vi "octave_var.vi"() -> ()   [LabVIEW 2011]
doc: "Octave interface global variables."
panel:
  out "proc handle":u32[](array[numeric])
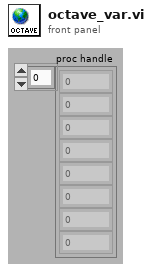
[diagram p1: front panel]
diagram:
